vi "TLB Native Dynamic Events ver 0.06a.vi"() -> ()   [LabVIEW 2018]
uses:
  Labview Training Phase 2/Enum Controls/States for Action Engine.ctl
  Type def/TLB event states.ctl
  Type def/TLB MHL States.ctl
  <vilib>/Studica/Studica Toolkit/Background/I2C Channel.ctl
  <vilib>/Studica/Studica Toolkit/NavX/NavX.lvlib
  <vilib>/myRIO/Common/Instrument Driver Framework/myRIO v1.0/AI/typedefs/AI Channels Enum.ctl
  <vilib>/myRIO/Common/Instrument Driver Framework/myRIO v1.0/AI/typedefs/AI Channels List.ctl
  Type def/Type def.ctl
  Type def/Motor Control Cluster.ctl
  <vilib>/Studica/Studica Blackhawk/Blackhawk.lvlib
  <vilib>/vision/driver/NI_Vision_Acquisition_Software.lvlib
  <vilib>/userdefined/High Color/IMAQdx.ctl
  <vilib>/vision/driver/IMAQdx.llb/IMAQdx Buffer Number Mode.ctl
  <vilib>/vision/driver/IMAQdx.llb/IMAQdx Acquisition Mode.ctl
  Underlying VI's/Webcam FGV Low level ver/State control.ctl
  <vilib>/Studica/Studica Toolkit/Background/Mxp Selection.ctl
  <vilib>/ptbypt/NI_PtbyPt.lvlib
panel:
  in  "wTargetSpeed":dbl(slide) scale=-1.0..1.0
  in  "yTargetSpeed":dbl(slide) scale=-1.0..1.0
  in  "xTargetSpeed":dbl(slide) scale=-1.0..1.0
  out "Speed":T1
  out "Distance":T2
  out "Blackhawk loop":i32
  out "NavX Loop":i32
  out "Sensor Loop":i32
  out "User event loop":i32
  out "Event handling loop":i32
  out "Main Loop":i32
  out "Status loop":i32
  out "Waveform Chart 3":dbl(graph)
  out "Waveform Chart 2":dbl(graph)
  out "Waveform Chart":dbl(graph)
  out "L/R average":fxp<+,64,64>
  out "Right Ultrasonic":fxp<+,64,16>
  out "Left Ultrasonic":fxp<+,64,16>
  out "Object detection count":T3
  out "Camera error":errorcluster
  out "Right IR Sensor":dbl
  out "Left IR Sensor":dbl
  in  "Servo Angle":u8(slide) scale=0.0..180.0
  in  "On/Off":bool
  out "Blackhawk error":errorcluster
  out "Value Read":bool
  out "Image Out":T4(plugin-control)
  out "element":T5
  out "Action Queue Items":i32
  out "State Logic Queue Items":i32
  out "Action Queues items":string[](array[string])=["Hardware reset", "Software reset", ""]
  out "State logic":T6=enum."Task 2"
  out "Action State":string
  in  "Tasks Selector":string(combo)="Default"
  out "Yaw":dbl
  out "NavX Info Out":T8
  out "LinearAcceleration":T9
  out "Displacement":T10
  out "YRPHfH":T11
  out "Object detected":bool
  in  "NavX Zero Yaw":bool
  in  "Return to IDLE":bool
  in  "Reset Encoders":bool
  in  "Stop Queue":bool
  in  "Start Task":bool
  # "Camera Status Loop"
  # "TLB FRAMEWORK STATUS"
  # "Test Programme written by Calvin Loke    Dated: 28 Aug 2019\nTest Programme revised by Dr Alex See   Dated 30 Aug 2019\n\nProgramme version:   TLB Native Dynamic Events ver 0.04b.vi"
  # "Sequence of Actions"
  # "Continuous (Repeated)"
  # "Motor Control Loop"
  # "Sensor data"
  # "Blackhawk status"
  # "System Health Status Update"
  # "NAVX Control Loop"
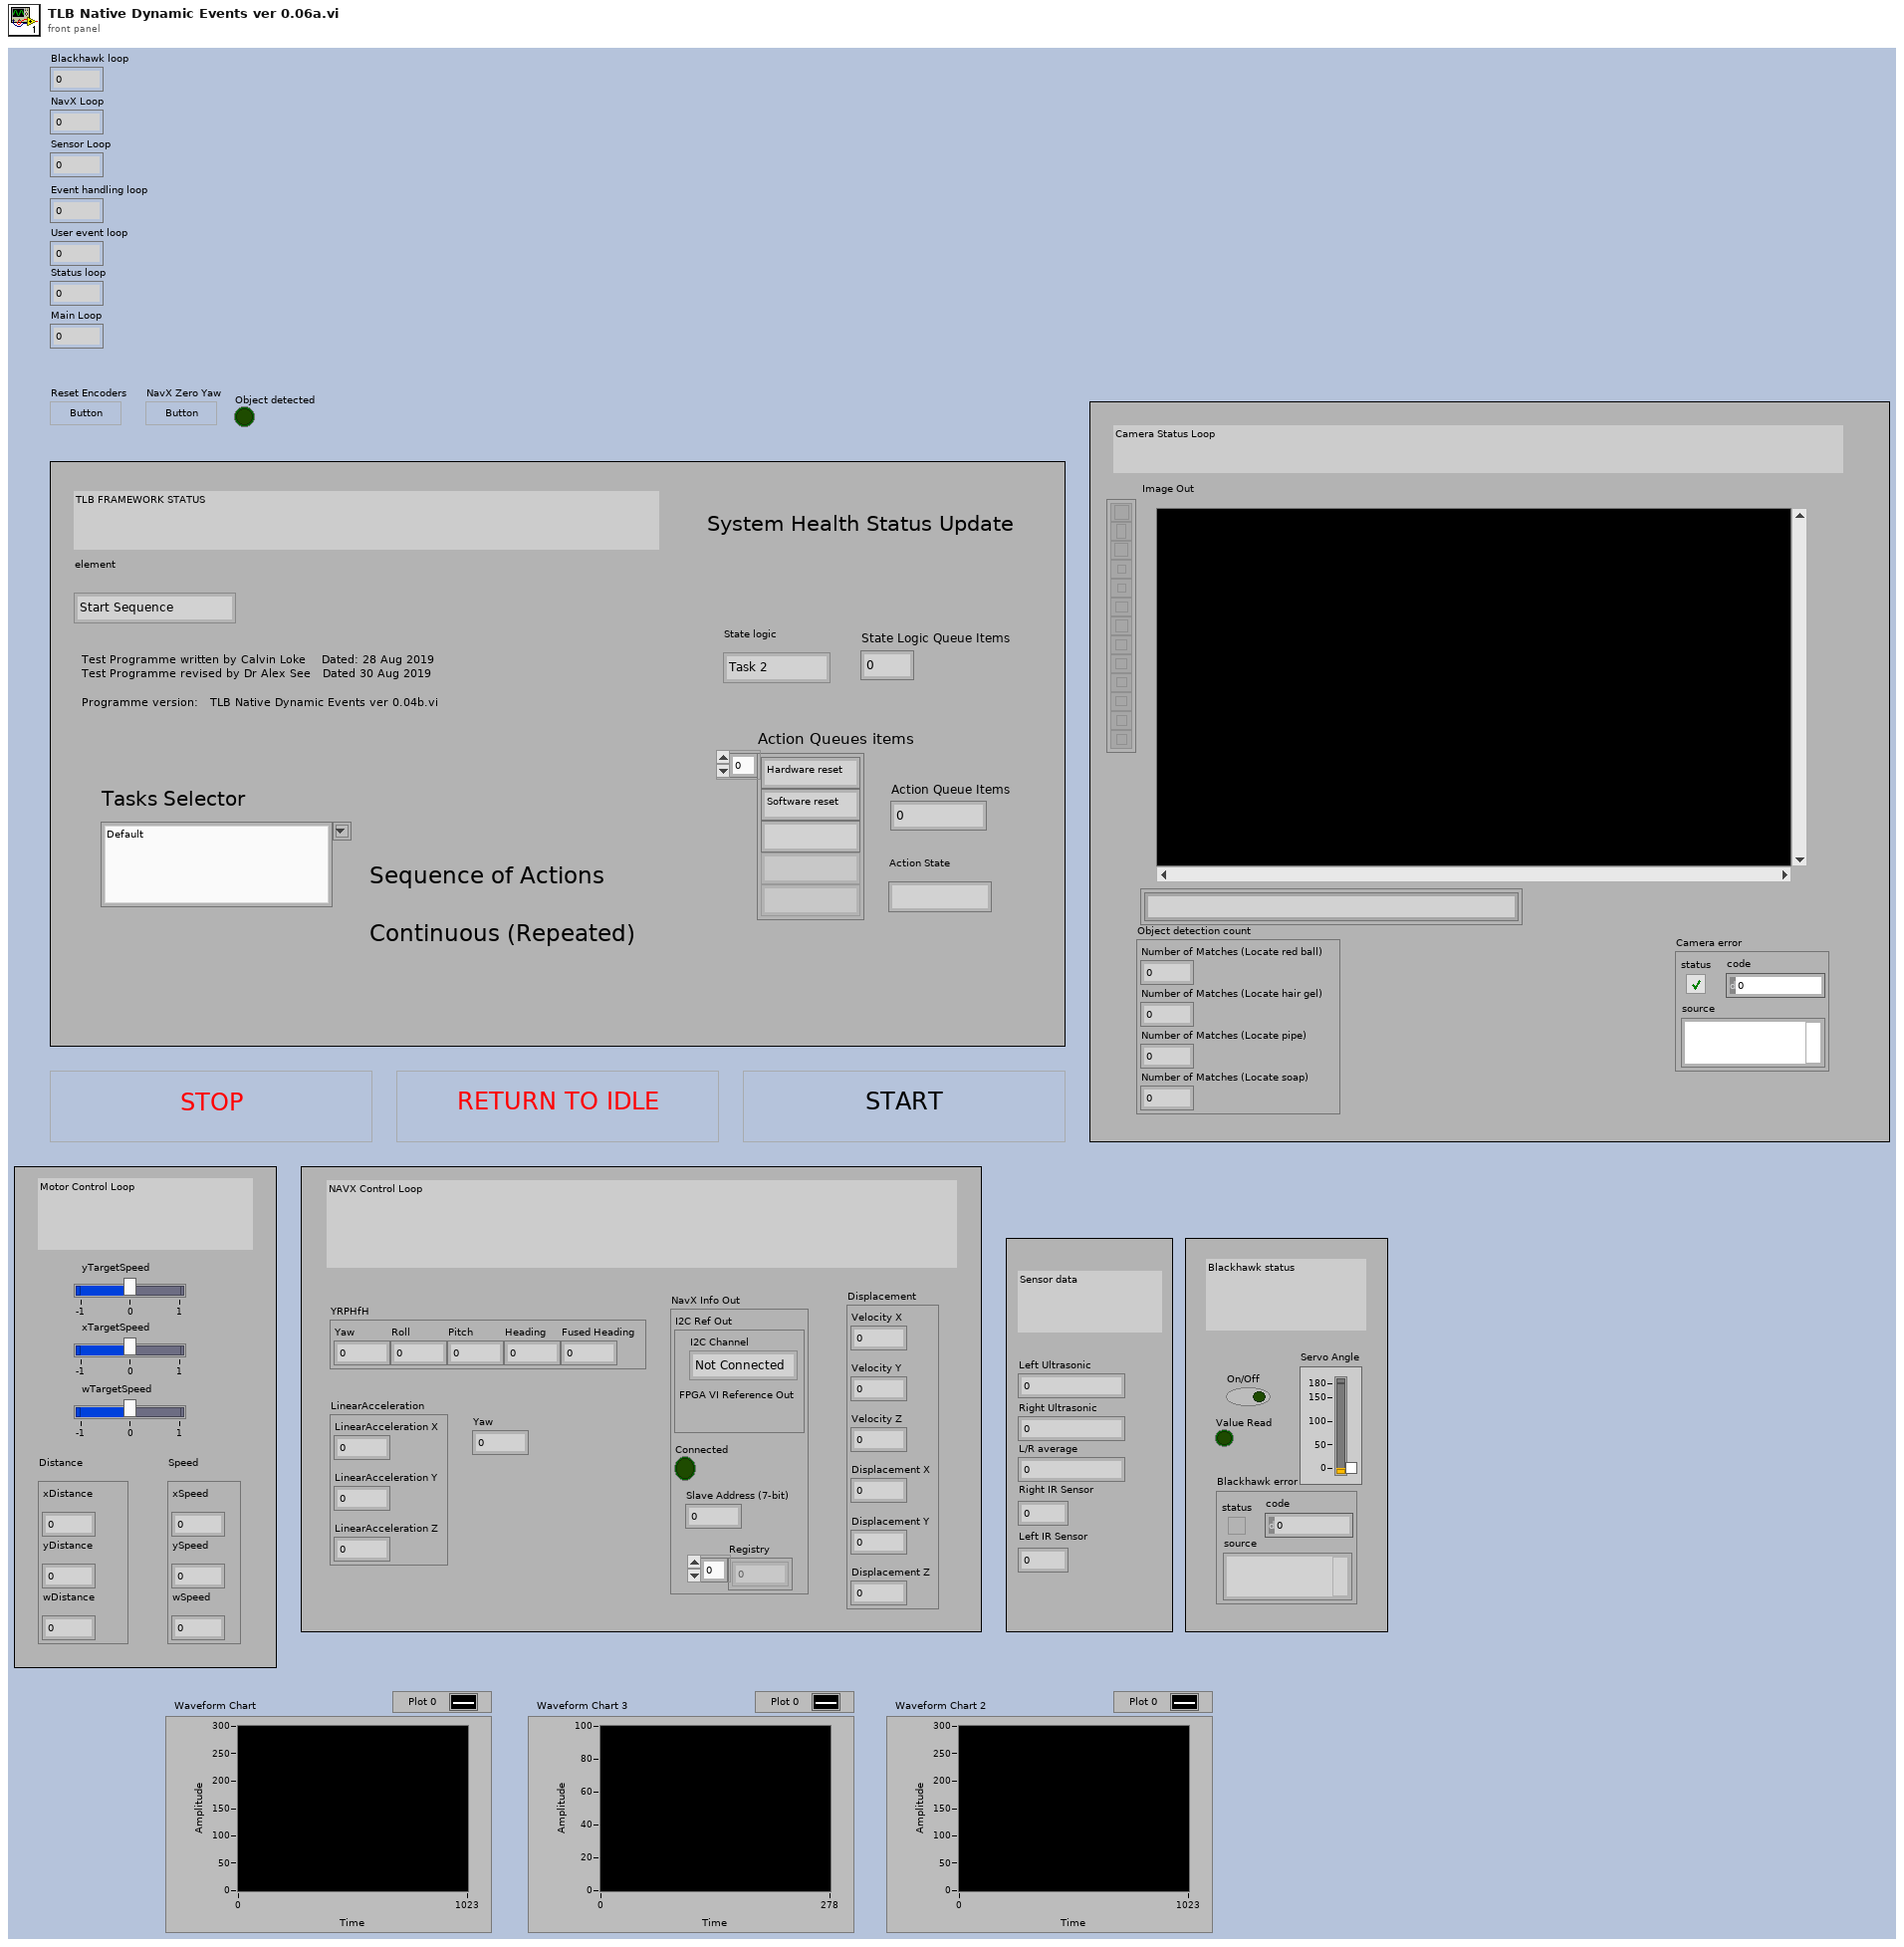
[diagram p1: front panel]
types:
  T1 = cluster{"xSpeed":dbl, "ySpeed":dbl, "wSpeed":dbl}
  T2 = cluster{"xDistance":dbl, "yDistance":dbl, "wDistance":dbl}
  T3 = cluster{"Number of Matches (Locate red ball)":i32, "Number of Matches (Locate hair gel)":i32, "Number of Matches (Locate pipe)":i32, "Number of Matches (Locate soap)":i32}
  T4 = typedef "IMAQ Image.ctl" = refnum<image>
  T5 = typedef "TLB event states.ctl" = enum16{"Start Sequence", "Exit", "Start Task 1", "Start Task 2", "Start Task 3", "Start Task 4", "Camera vision", "Wall follow mode", "Idle", "Start Drive Straight"}
  T6 = typedef "TLB MHL States.ctl" = enum16{"None", "Startup", "Idle", "Processing", "Shutdown", "Reset", "Task 1", "Task 2", "Task 3", "Task 4", "Task 4a", "Task 4b", "Task 4c", "Task 4d", "Task 4e", "Task 4f", "Task 4g", "Task 4h", "Acquire image", "Wall follow mode", "Autodrive", "Autodrive a"}
  T7 = typedef "I2C Channel.ctl" = enum16{"Not Connected", "A", "B"}
  T8 = cluster{"I2C Ref Out":cluster{"I2C Channel":T7, "FPGA VI Reference Out":refnum<k20>}, "Connected":bool, "Slave Address (7-bit)":u8, "Registry":u8[]}
  T9 = cluster{"LinearAcceleration X":dbl, "LinearAcceleration Y":dbl, "LinearAcceleration Z":dbl}
  T10 = cluster{"Velocity X":dbl, "Velocity Y":dbl, "Velocity Z":dbl, "Displacement X":dbl, "Displacement Y":dbl, "Displacement Z":dbl}
  T11 = cluster{"Yaw":dbl, "Roll":dbl, "Pitch":dbl, "Heading":dbl, "Fused Heading":dbl}
  T12 = typedef "States for Action Engine.ctl" = enum16{"Initialize", "Write", "Read"}
  T13 = typedef "Motor Control Cluster.ctl" = cluster{"Vx":dbl, "Vy":dbl, "Vw":dbl}
  T14 = typedef "Type def.ctl" = cluster{"Front Ultrasonic Obstruct":bool, "Left Ultrasonic Obstruct":bool, "Right Ultrasonic Obstruct ":bool}
  T15 = typedef "NI_Vision_Acquisition_Software.lvlib/IMAQdx Acquisition Mode.ctl" = enum32{"One Shot", "Continuous"}
  T16 = typedef "IMAQdx.ctl" = refnum<k21>
  T17 = typedef "NI_Vision_Acquisition_Software.lvlib/IMAQdx Buffer Number Mode.ctl" = enum32{"Next", "Last", "Buffer Number", "Every", "Last New"}
  T18 = typedef "Mxp Selection.ctl" = enum16{"MXP A", "MXP B"}
  T19 = typedef "State control.ctl" = enum16{"Initialise", "Start camera", "Continuous Acquisition ", "Stop camera", "Dispose all"}
  T20 = typedef "AI Channels List.ctl" = T21[]
  T21 = typedef "AI Channels Enum.ctl" = enum16{"Not Connected", "AudioIn/Left", "AudioIn/Right", "C/AI0", "C/AI1", "A/AI0", "A/AI1", "A/AI2", "A/AI3", "A/AI4", "A/AI5", "A/AI6", "A/AI7", "B/AI0", "B/AI1", "B/AI2", "B/AI3", "B/AI4", "B/AI5", "B/AI6", "B/AI7", "AI/AI0", "AI/AI1", "AI/AI2", "AI/AI3", "A/AI0 (DIFF)", "A/AI1 (DIFF)", "A/AI2 (DIFF)", "A/AI3 (DIFF)", "B/AI0 (DIFF)", "B/AI1 (DIFF)", "B/AI2 (DIFF)", "B/AI3 (DIFF)"}
  T22 = cluster{"I2C Channel":T7, "FPGA VI Reference Out":refnum<k20>}
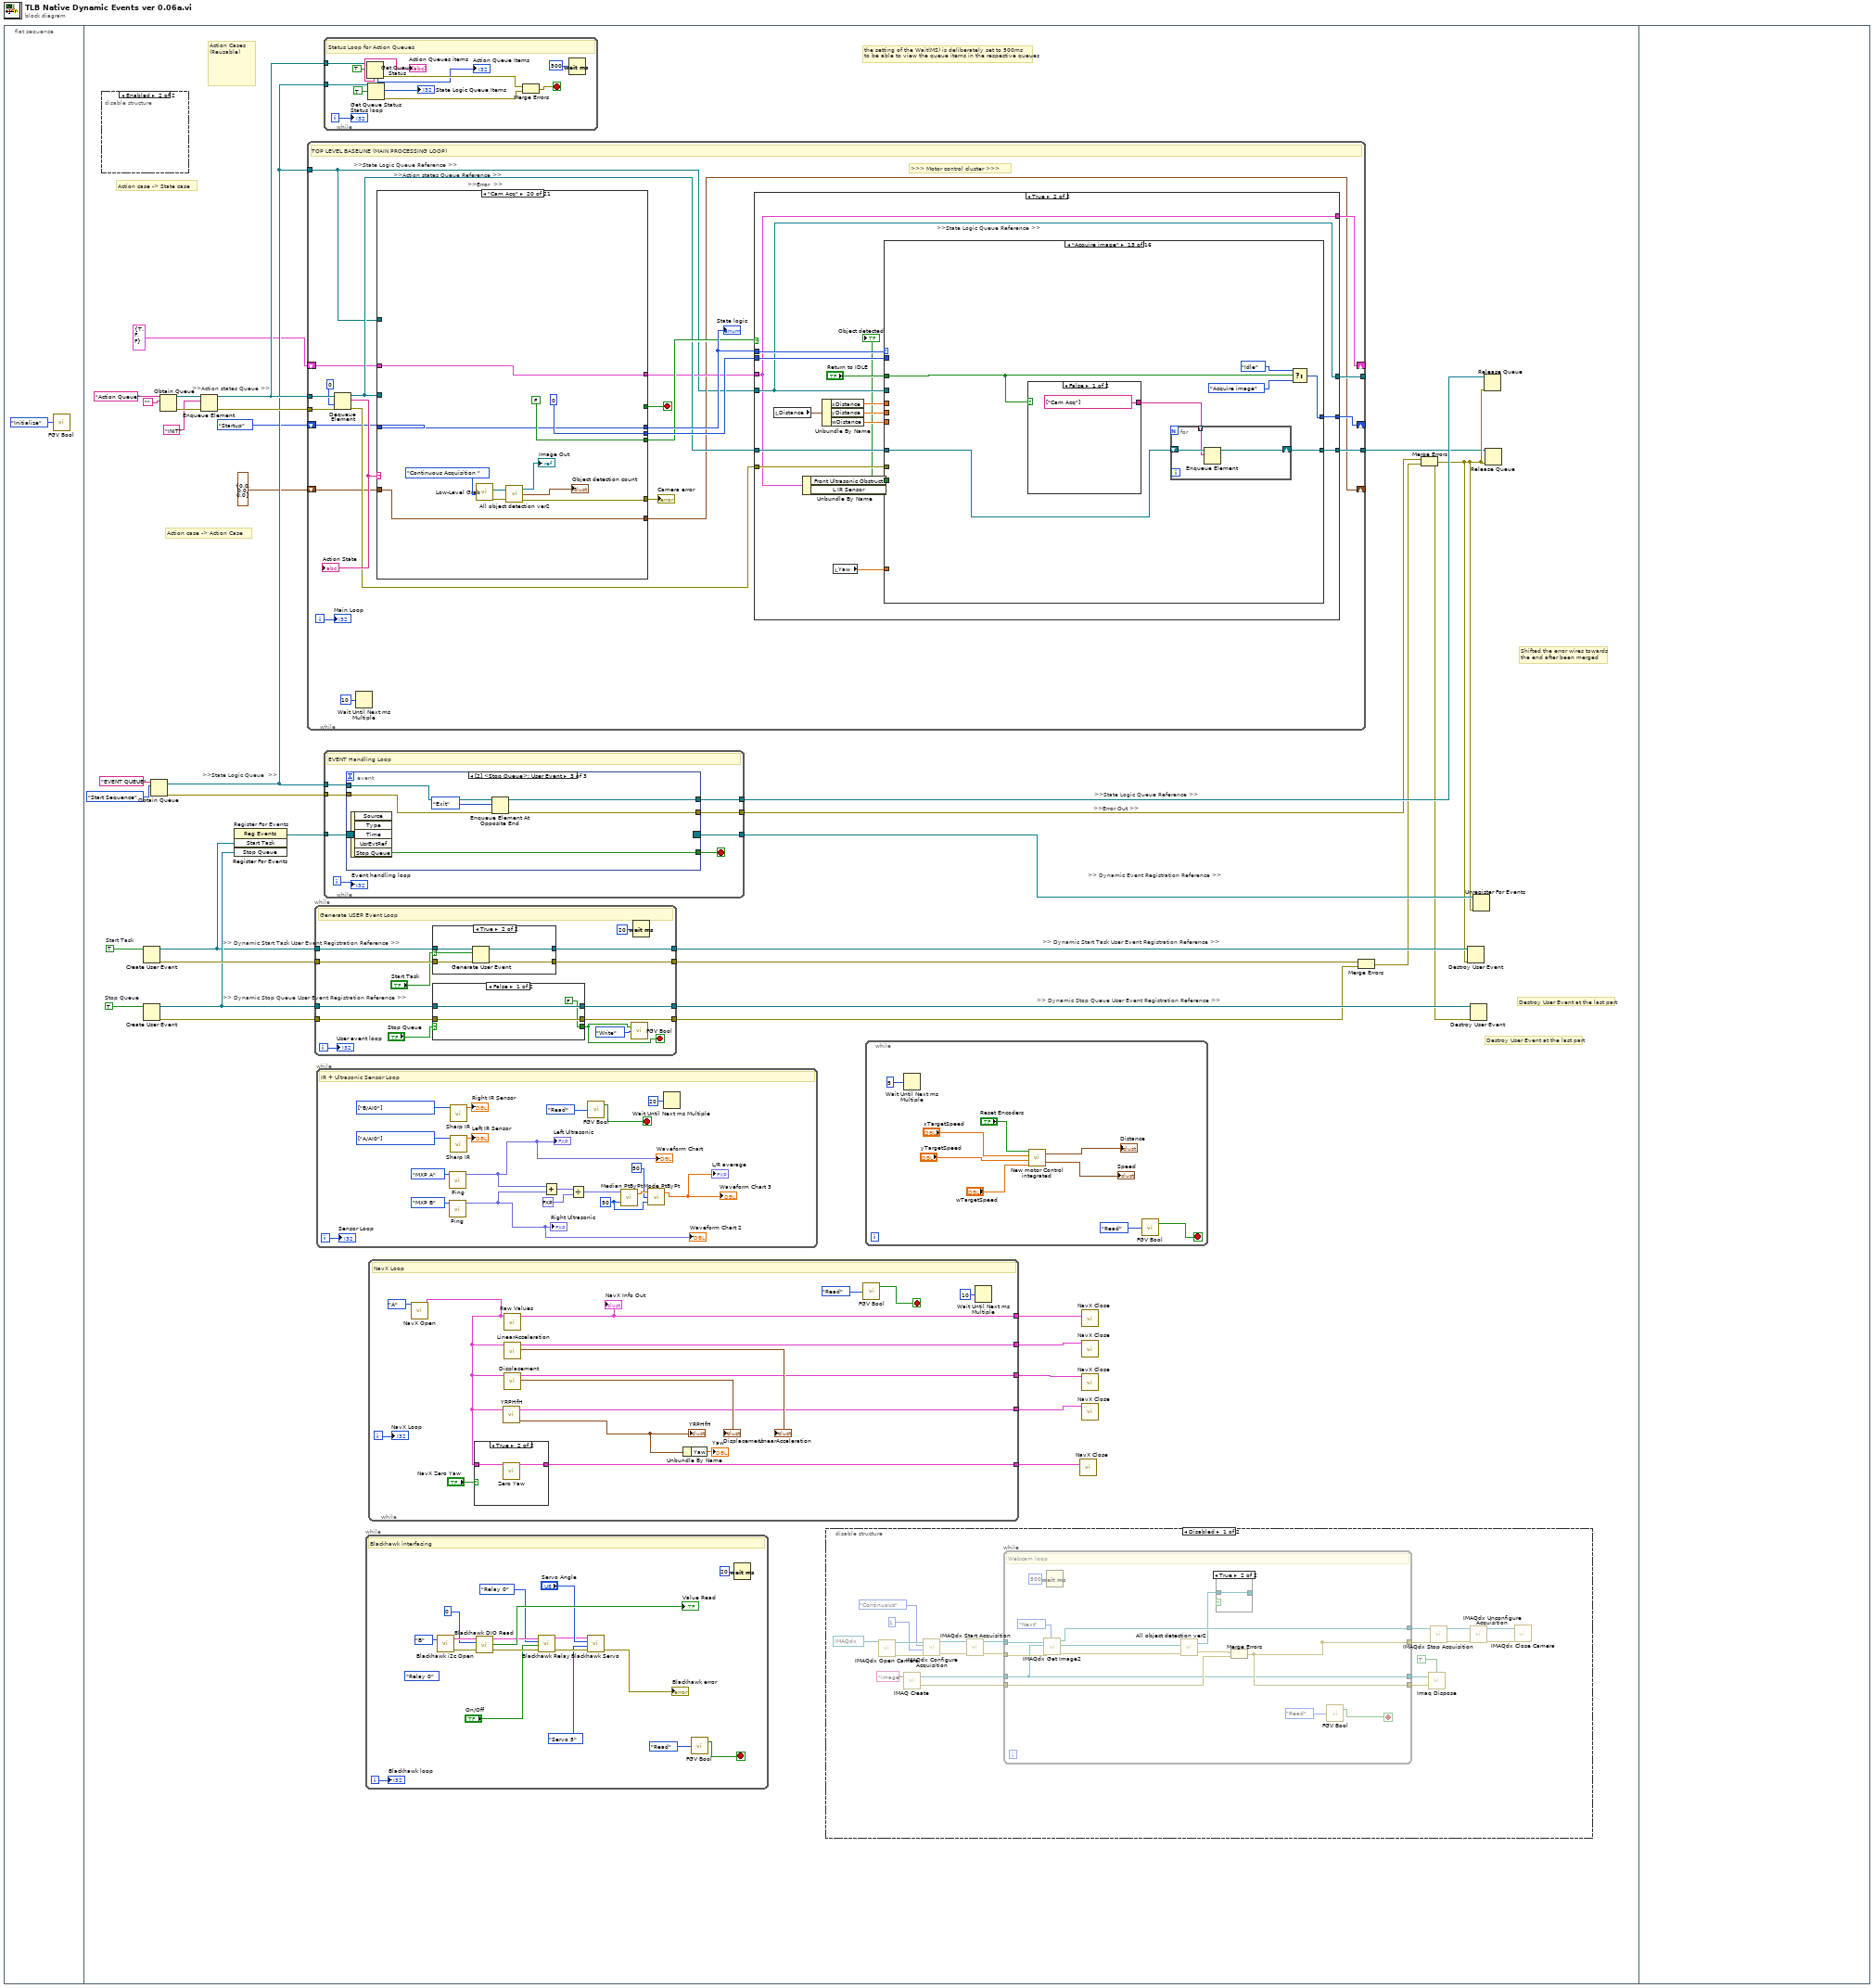
[diagram p0: block diagram]
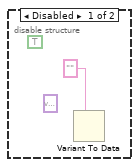
[diagram p5: hidden frame]
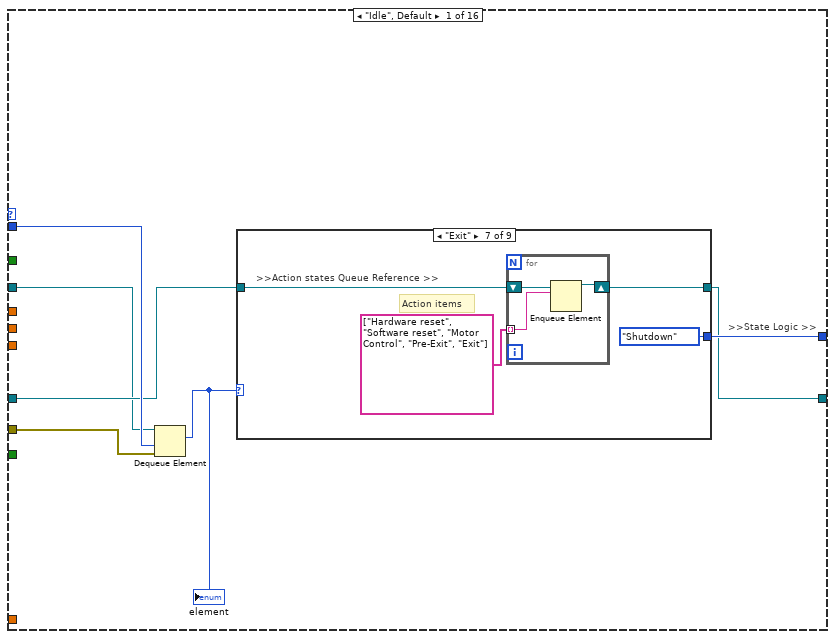
[diagram p7: hidden frame]
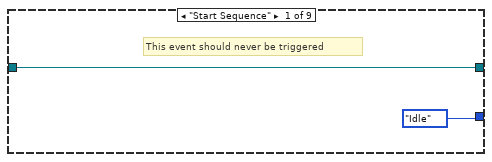
[diagram p8: hidden frame]
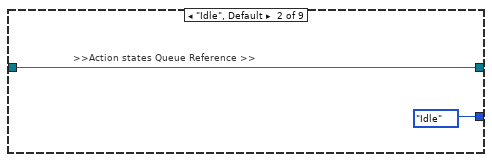
[diagram p9: hidden frame]
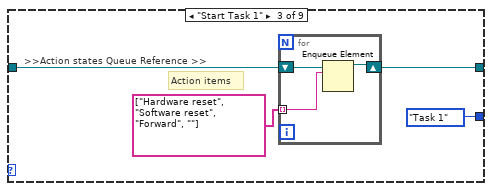
[diagram p10: hidden frame]
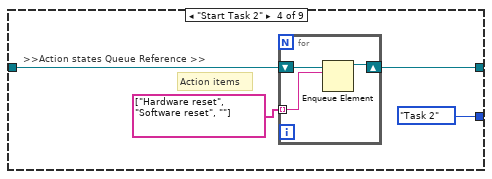
[diagram p11: hidden frame]
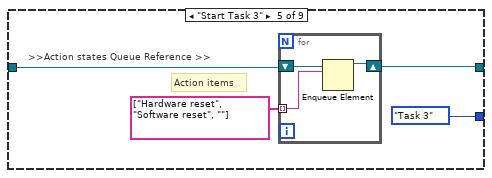
[diagram p12: hidden frame]
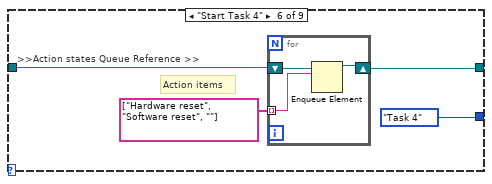
[diagram p13: hidden frame]
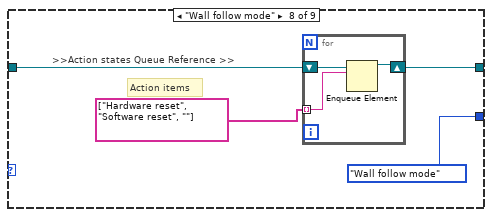
[diagram p14: hidden frame]
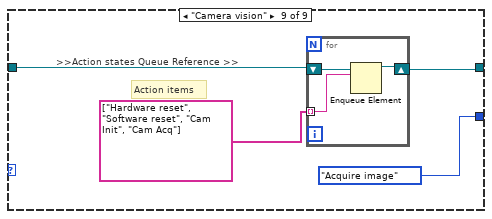
[diagram p15: hidden frame]
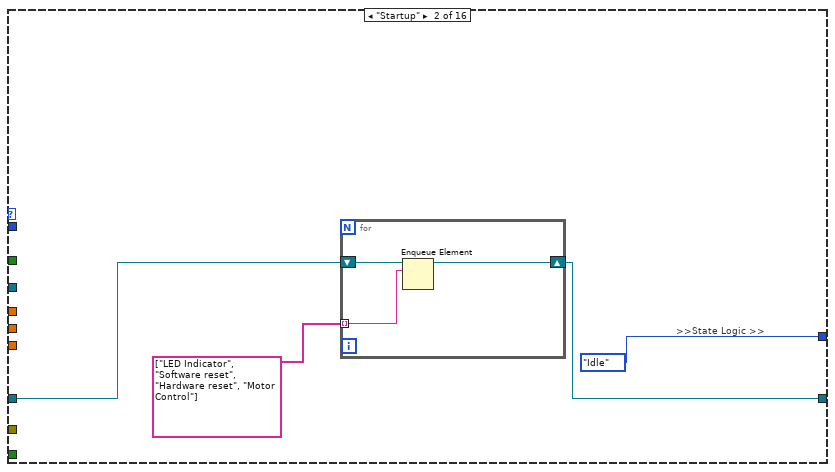
[diagram p16: hidden frame]
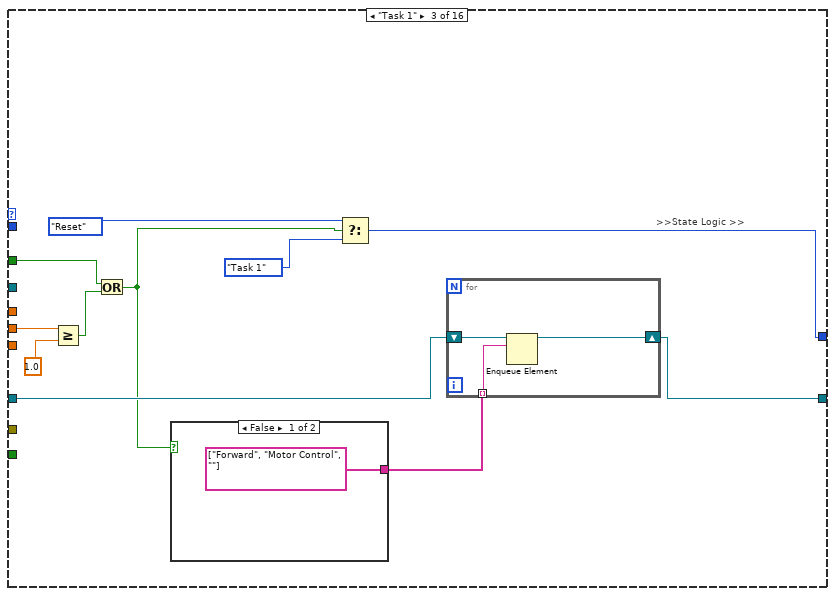
[diagram p17: hidden frame]
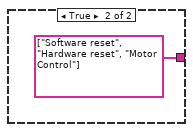
[diagram p18: hidden frame]
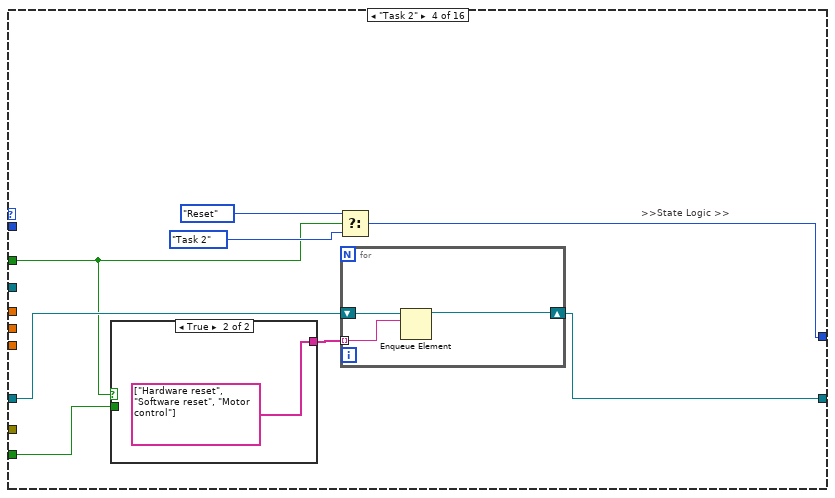
[diagram p19: hidden frame]
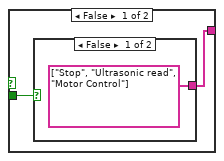
[diagram p20: hidden frame]
diagram:
  n1 = flat-sequence {
    frame #0 {
      n2 = call "FGV Bool.vi"("Init/Read/Write State"=States_for_Action_Engine."Initialize") -> ()  [unwired: 2 in, 2 out]
    }
    frame #1 {
      w37 = TRUE  # Stop Queue
      w36 = TRUE  # Start Task
      # "Action case -> Action Case"
      # "Action case -> State case"
      # "the setting of the Wait(MS) is deliberately set to 500ms\nto be able to view the queue items in the respective queues"
      # "Action Cases\n(Reusable)"
      # ">>Error Out >>"
      # ">> Dynamic Stop Queue User Event Registration Reference >>"
      # ">> Dynamic Start Task User Event Registration Reference >>"
      # ">> Dynamic Stop Queue User Event Registration Reference >>"
      # ">> Dynamic Start Task User Event Registration Reference >>"
      # ">> Dynamic Event Registration Reference >>"
      # ">>Action states Queue >>"
      # ">>State Logic Queue  >>"
      # ">>State Logic Queue Reference >>"
      # "Destroy User Event at the last part"
      # "Destroy User Event at the last part"
      # "Shifted the error wires towards\nthe end after been merged"
      n3 = disable-structure shown="Enabled" {
        frame Disabled {
          (unwired) variant
          (unwired) TRUE
          n4 = Variant To Data(type="") -> ()  [unwired: 2 in, 2 out]
        }
        frame Enabled {
        }
      }
      n5 = Create User Event(user event datatype=w36) -> (user event=w28:refnum<user-event>, error out=w33:errorcluster)  [unwired: 1 in]
      n6 = Create User Event(user event datatype=w37) -> (user event=w29:refnum<user-event>, error out=w32:errorcluster)  [unwired: 1 in]
      n7 = Obtain Queue(name (unnamed)="EVENT QUEUE", element data type=TLB_event_states."Start Sequence" ("Enum")) -> (queue out=w13:refnum<queue>, error out=w19:errorcluster)  [unwired: 3 in, 1 out]
      n8 = Obtain Queue(name (unnamed)="Action Queue", element data type="") -> (queue out=w22:refnum<queue>, error out=w18:errorcluster)  [unwired: 3 in, 1 out]
      n9 = Enqueue Element(queue=w22, element="INIT", error in (no error)=w18) -> (queue out=w14:refnum<queue>, error out=w17:errorcluster)  [unwired: 1 in, 1 out]
      n10 = register-events "Register For Events"(w28, w29) -> (reference out=w27:refnum<event-registration>)  [unwired: 2 in, 1 out]
      n11 = while {
        tunnel: w13 -> [w154]
        shift-right: [w169] -> _
        shift-left: TLB_MHL_States."Startup" ("Enum") -> [w162]
        tunnel: w14 -> [w174]
        tunnel: w17 -> [w172]
        tunnel: [w171] -> _
        tunnel: [w170] -> w11
        shift-right: [w159] -> _
        shift-left: T14 {"Front Ultrasonic Obstruct"=TRUE, "Left Ultrasonic Obstruct"=FALSE, "Right Ultrasonic Obstruct "=FALSE} -> [w161]
        shift-right: [w157] -> _
        shift-left: T13 {"Vx"=0.0, "Vy"=0.0, "Vw"=0.0} -> [w158]
        i -> [w155]
        stop <- w167 stop-if-true
        # ">>> Motor control cluster >>>"
        # ">>Error  >>"
        # ">>Action states Queue Reference >>"
        # ">>State Logic Queue Reference >>"
        # "TOP LEVEL BASELINE (MAIN PROCESSING LOOP)"
        n12 = Dequeue Element(queue=w174, timeout in ms (-1)=0, error in (no error)=w172) -> (queue out=w163:refnum<queue>, element=w173:string, error out=w164:errorcluster)  [unwired: 1 out]
        "Action State" <- w173
        n13 = Wait Until Next ms Multiple(millisecond multiple=u32 10) -> ()  [unwired: 1 out]
        n14 = case shown="\"Cam Acq\"" w173 {
          tunnel: [w420 w437 w442 w450 w459 w469 w478 w485 w496 w504 w512 w522 w532 TLB_MHL_States."Shutdown" ("Enum") w542 w552 w556 w570 w582 w591 w605] -> w175
          tunnel: [w427 0 0 0 0 0 0 0 0 0 0 0 0 0 0 0 0 0 0 0 0] -> w168
          tunnel: [_ _ _ _ _ _ _ _ _ _ _ _ _ TRUE _ _ _ _ _ _ _] -> w167
          tunnel: [TRUE FALSE FALSE FALSE FALSE FALSE FALSE FALSE FALSE FALSE FALSE FALSE FALSE FALSE FALSE FALSE FALSE FALSE FALSE FALSE FALSE] -> w166
          tunnel: w163 -> [w419 _ _ _ _ _ _ _ _ _ _ _ _ _ _ _ _ _ _ _ _]
          tunnel: w162 -> [w421 w437 w442 w450 w459 w469 w478 w485 w496 w504 w512 w522 w532 _ w542 w552 w556 w570 w582 w591 w605]
          tunnel: w161 -> [w425 w434 w439 w446 w455 w464 w473 w482 w491 w500 w513 w519 w527 w534 w543 w551 w559 w571 w583 w590 w601]
          tunnel: [w425 w434 w439 w446 w455 w464 w473 w482 w491 w500 w513 w518 w527 w534 w543 w548 w558 w571 w583 w590 w601] -> w160
          tunnel: w158 -> [w424 w433 w438 w444 w453 w462 w472 w480 w490 w498 w509 w516 w526 w533 w539 w545 w553 w562 w581 w594 w602]
          tunnel: [w424 w433 w438 w445 w454 w463 w471 w481 w489 w499 w509 w516 w524 w533 w539 w545 w553 w563 w581 w594 w602] -> w157
          tunnel: [_ _ _ _ _ _ _ _ _ _ _ _ _ _ _ _ _ _ w572 w586 w595] -> w156
          tunnel: w154 -> [w423 _ _ _ _ _ _ _ _ _ _ _ _ _ _ _ _ _ _ _ _]
          frame "No action", Default {
            n15 = Get Queue Status(queue=w423) -> (error out=w422:errorcluster)  [unwired: 2 in, 7 out]
            n16 = case shown="Error" w422 {
              tunnel: w421 -> [w428 _]
              tunnel: [w428 TLB_MHL_States."Shutdown" ("Enum")] -> w420
              tunnel: w419 -> [_ _]
              frame No Error {
              }
              frame Error {
              }
            }
            n17 = case shown="\"Startup\", Default" w421 {
              tunnel: [0 100] -> w427
              frame "Startup", Default {
              }
              frame "Idle" {
              }
            }
          }
          frame "Init" {
            # ">>State Logic  >>"
            n18 = local write "Servo Angle"(u8 90 ("Servo Angle")) -> ()
          }
          frame "LED Indicator" {
          }
          frame "Forward" {
            n19 = local write "NavX Zero Yaw"(FALSE ("NavX Zero Yaw")) -> ()
            n20 = local write "Reset Encoders"(FALSE ("Reset Encoder 0")) -> ()
            n21 = Bundle By Name(cluster=w444, "Vy"=0.6) -> (w445:T13)
          }
          frame "Reverse" {
            n22 = local write "NavX Zero Yaw"(FALSE ("NavX Zero Yaw")) -> ()
            n23 = local write "Reset Encoders"(FALSE ("Reset Encoder 0")) -> ()
            n24 = Bundle By Name(cluster=w453, "Vy"=-0.6) -> (w454:T13)
          }
          frame "Right" {
            n25 = local write "NavX Zero Yaw"(FALSE ("NavX Zero Yaw")) -> ()
            n26 = local write "Reset Encoders"(FALSE ("Reset Encoder 0")) -> ()
            n27 = Bundle By Name(cluster=w462, "Vx"=0.6) -> (w463:T13)
          }
          frame "Left" {
            n28 = Bundle By Name(cluster=w472, "Vx"=-0.6) -> (w471:T13)
            n29 = local write "NavX Zero Yaw"(FALSE ("NavX Zero Yaw")) -> ()
            n30 = local write "Reset Encoders"(FALSE ("Reset Encoder 0")) -> ()
          }
          frame "Rotate CW" {
            n31 = local write "NavX Zero Yaw"(FALSE ("NavX Zero Yaw")) -> ()
            n32 = local write "Reset Encoders"(FALSE ("Reset Encoder 0")) -> ()
            n33 = Bundle By Name(cluster=w480, "Vw"=-0.3) -> (w481:T13)
          }
          frame "Rotate ACW" {
            n34 = local write "Reset Encoders"(FALSE ("Reset Encoder 0")) -> ()
            n35 = local write "NavX Zero Yaw"(FALSE ("NavX Zero Yaw")) -> ()
            n36 = Bundle By Name(cluster=w490, "Vw"=0.15) -> (w489:T13)
          }
          frame "Stop" {
            w497 = 0.0
            n37 = local write "NavX Zero Yaw"(FALSE ("NavX Zero Yaw")) -> ()
            n38 = local write "Reset Encoders"(FALSE ("Reset Encoder 0")) -> ()
            n39 = Bundle By Name(cluster=w498, "Vx"=w497, "Vy"=w497, "Vw"=w497) -> (w499:T13)
          }
          frame "Motor control" {
            # "Replace with FGV"
            n40 = Unbundle By Name(w509) -> ("Vx"=w508:dbl, "Vy"=w507:dbl, "Vw"=w506:dbl)
            n41 = local write "xTargetSpeed"(w508) -> ()
            n42 = local write "yTargetSpeed"(w507) -> ()
            n43 = local write "wTargetSpeed"(w506) -> ()
          }
          frame "Software reset" {
            w517 = FALSE ("NavX Zero Yaw")
            n44 = Wait (ms)(milliseconds to wait=u32 20) -> ()  [unwired: 1 out]
            n45 = local write "NavX Zero Yaw"(w517) -> ()
            n46 = Bundle By Name(cluster=w519, "Front Ultrasonic Obstruct"=w517, "L IR Sensor"=0.0) -> (w518:T14)
          }
          frame "Hardware reset" {
            w525 = 0.0
            n47 = Wait (ms)(milliseconds to wait=u32 20) -> ()  [unwired: 1 out]
            n48 = local write "NavX Zero Yaw"(TRUE ("NavX Zero Yaw")) -> ()
            n49 = local write "Reset Encoders"(TRUE ("Reset Encoder 0")) -> ()
            n50 = Bundle By Name(cluster=w526, "Vx"=w525, "Vy"=w525, "Vw"=w525) -> (w524:T13)
          }
          frame "Exit" {
          }
          frame "Pre-Exit" {
          }
          frame "Ultrasonic read" {
            # "Object detection"
            n51 = local read "L/R average"() -> (w544:fxp<+,64,64>)
            n52 = Less Or Equal?(x=w544, y=35.0) -> (x <= y?=w546:bool)
            n53 = Bundle By Name(cluster=w551, "Front Ultrasonic Obstruct"=w546) -> (w548:T14)
          }
          frame "IR Sensor Read" {
            n54 = local read "Left IR Sensor"() -> (w557:dbl)
            n55 = Bundle By Name(cluster=w559, "L IR Sensor"=w557) -> (w558:T14)
          }
          frame "Calculate" {
            n56 = Unbundle By Name(w571) -> ("L IR Sensor"=w567:dbl)
            n57 = Subtract(x=w567, y=20.0) -> (x-y=w565:dbl)
            n58 = Multiply(x=w565, y=0.01) -> (x*y=w561:dbl)
            n59 = Bundle By Name(cluster=w562, "Vy"=0.4, "Vw"=w561) -> (w563:T13)
          }
          frame "Cam Init" {
            n60 = call "Low-Level Grab.vi"("States"=State_control."Initialise", "Session In"=T16 "cam1") -> ("error out"=w573:errorcluster, "Session Out"=w574:T16)  [unwired: 7 in, 1 out]
            n61 = call "Low-Level Grab.vi"("error in (no error)"=w573, "States"=State_control."Start camera", "Session In"=w574) -> ("error out"=w572:errorcluster)  [unwired: 6 in, 2 out]
            n62 = local write "Servo Angle"(u8 170 ("Servo Angle")) -> ()
          }
          frame "Cam Acq" {
            n63 = call "Low-Level Grab.vi"("States"=State_control."Continuous Acquisition ") -> ("error out"=w587:errorcluster, "Image Out"=w588:T4)  [unwired: 8 in, 1 out]
            n64 = call "All object detection ver2.vi"("Image In"=w588, "error in"=w587) -> ("Image Out"=→"Image Out":T4, "Object detection count"=→"Object detection count":T3, "error out"=w586:errorcluster)
          }
          frame "Cam Exit" {
            n65 = call "Low-Level Grab.vi"("States"=State_control."Stop camera") -> ("error out"=w596:errorcluster, "Session Out"=w598:T16)  [unwired: 8 in, 1 out]
            n66 = local write "Servo Angle"(u8 90 ("Servo Angle")) -> ()
            n67 = call "Low-Level Grab.vi"("error in (no error)"=w596, "States"=State_control."Dispose all", "Session In"=w598) -> ("error out"=w595:errorcluster)  [unwired: 6 in, 2 out]
          }
        }
        "State logic" <- w175
        "Camera error" <- w156
        n68 = case shown="True" w166 {
          tunnel: w175 -> [w178 w194]
          tunnel: w154 -> [w179 w188]
          tunnel: w163 -> [w177 w193]
          tunnel: [w179 w188] -> w171
          tunnel: [w177 w192] -> w170
          tunnel: [w178 w191] -> w169
          tunnel: w164 -> [_ w190]
          tunnel: w168 -> [_ w189]
          tunnel: w160 -> [w176 w181]
          tunnel: [w176 w181] -> w159
          frame False {
          }
          frame True {
            # ">>State Logic Queue Reference >>"
            n69 = local read "Distance"() -> (w180:T2)
            n70 = Unbundle By Name(w181) -> ("Front Ultrasonic Obstruct"=w182:bool)  [unwired: 1 out]
            "Object detected" <- w182
            n71 = Unbundle By Name(w180) -> ("xDistance"=w184:dbl, "yDistance"=w186:dbl, "wDistance"=w185:dbl)
            n72 = local read "Yaw"() -> (w183:dbl)
            n73 = case shown="\"Acquire image\"" w194 {
              tunnel: w188 -> [w195 _ _ _ _ _ _ _ _ _ _ _ _ _ _ _]
              tunnel: w193 -> [w197 w256 w268 w281 w303 w312 w326 w341 w354 w367 w378 w386 w399 w408 w411 w417]
              tunnel: [w196 w255 w267 w282 w302 w313 w325 w340 w353 w366 w377 w387 w398 w408 w410 w417] -> w192
              tunnel: [w200 TLB_MHL_States."Idle" ("Enum") w270 w283 w299 w316 w328 w339 w355 w365 TLB_MHL_States."Idle" ("Enum") w389 w397 TLB_MHL_States."Reset" ("Enum") TLB_MHL_States."Shutdown" ("Enum") TLB_MHL_States."Reset" ("Enum")] -> w191
              tunnel: w190 -> [w198 _ _ _ _ _ _ _ _ _ _ _ _ _ _ _]
              tunnel: w189 -> [w199 _ _ _ _ _ _ _ _ _ _ _ _ _ _ _]
              tunnel: "Return to IDLE" -> [_ _ w265 w280 w297 _ _ _ _ _ _ w384 w396 _ _ _]
              tunnel: w186 -> [_ _ w262 _ _ _ w322 w336 _ _ _ _ _ _ _ _]
              tunnel: w185 -> [_ _ _ _ w294 _ _ _ _ _ _ _ _ _ _ _]
              tunnel: w184 -> [_ _ _ _ _ _ _ _ w350 _ _ _ _ _ _ _]
              tunnel: w183 -> [_ _ _ _ _ _ _ _ _ _ _ _ _ _ _ _]
              tunnel: w182 -> [_ _ _ w278 _ w310 _ _ _ w364 _ _ _ _ _ _]
              frame "Idle", Default {
                # ">>State Logic >>"
                n74 = Dequeue Element(queue=w195, timeout in ms (-1)=w199, error in (no error)=w198) -> (element=w201:T5)  [unwired: 3 out]
                "element" <- w201
                n75 = case shown="\"Exit\"" w201 {
                  tunnel: [TLB_MHL_States."Idle" ("Enum") TLB_MHL_States."Idle" ("Enum") TLB_MHL_States."Task 1" ("Enum") TLB_MHL_States."Task 2" ("Enum") TLB_MHL_States."Task 3" ("Enum") TLB_MHL_States."Task 4" ("Enum") TLB_MHL_States."Shutdown" ("Enum") TLB_MHL_States."Wall follow mode" ("Enum") TLB_MHL_States."Acquire image" ("Enum")] -> w200
                  tunnel: [w203 w204 w208 w213 w222 w228 w234 w241 w249] -> w196
                  tunnel: w197 -> [w203 w204 w206 w214 w223 w229 w235 w242 w250]
                  frame "Start Sequence" {
                    # "This event should never be triggered"
                  }
                  frame "Idle", Default {
                    # ">>Action states Queue Reference >>"
                  }
                  frame "Start Task 1" {
                    # ">>Action states Queue Reference >>"
                    # "Action items"
                    n76 = for {
                      shift-right: [w212] -> w208
                      shift-left: w206 -> [w211]
                      tunnel: string[] ["Hardware reset", "Software reset", "Forward", ""] -> [w210] mode=indexing
                      n77 = Enqueue Element(queue=w211, element=w210) -> (queue out=w212:refnum<queue>)  [unwired: 2 in, 2 out]
                    }
                  }
                  frame "Start Task 2" {
                    # ">>Action states Queue Reference >>"
                    # "Action items"
                    n78 = for {
                      shift-right: [w219] -> w213
                      shift-left: w214 -> [w218]
                      tunnel: string[] ["Hardware reset", "Software reset", ""] -> [w217] mode=indexing
                      n79 = Enqueue Element(queue=w218, element=w217) -> (queue out=w219:refnum<queue>)  [unwired: 2 in, 2 out]
                    }
                  }
                  frame "Start Task 3" {
                    # ">>Action states Queue Reference >>"
                    # "Action items"
                    n80 = for {
                      shift-right: [w226] -> w222
                      shift-left: w223 -> [w225]
                      tunnel: string[] ["Hardware reset", "Software reset", ""] -> [w224] mode=indexing
                      n81 = Enqueue Element(queue=w225, element=w224) -> (queue out=w226:refnum<queue>)  [unwired: 2 in, 2 out]
                    }
                  }
                  frame "Start Task 4" {
                    # ">>Action states Queue Reference >>"
                    # "Action items"
                    n82 = for {
                      shift-right: [w233] -> w228
                      shift-left: w229 -> [w232]
                      tunnel: string[] ["Hardware reset", "Software reset", ""] -> [w231] mode=indexing
                      n83 = Enqueue Element(queue=w232, element=w231) -> (queue out=w233:refnum<queue>)  [unwired: 2 in, 2 out]
                    }
                  }
                  frame "Exit" {
                    # ">>Action states Queue Reference >>"
                    # "Action items"
                    n84 = for {
                      shift-right: [w240] -> w234
                      shift-left: w235 -> [w239]
                      tunnel: string[] ["Hardware reset", "Software reset", "Motor Control", "Pre-Exit", "Exit"] -> [w238] mode=indexing
                      n85 = Enqueue Element(queue=w239, element=w238) -> (queue out=w240:refnum<queue>)  [unwired: 2 in, 2 out]
                    }
                  }
                  frame "Wall follow mode" {
                    # ">>Action states Queue Reference >>"
                    # "Action items"
                    n86 = for {
                      shift-right: [w247] -> w241
                      shift-left: w242 -> [w246]
                      tunnel: string[] ["Hardware reset", "Software reset", ""] -> [w245] mode=indexing
                      n87 = Enqueue Element(queue=w246, element=w245) -> (queue out=w247:refnum<queue>)  [unwired: 2 in, 2 out]
                    }
                  }
                  frame "Camera vision" {
                    # ">>Action states Queue Reference >>"
                    # "Action items"
                    n88 = for {
                      shift-right: [w254] -> w249
                      shift-left: w250 -> [w253]
                      tunnel: string[] ["Hardware reset", "Software reset", "Cam Init", "Cam Acq"] -> [w252] mode=indexing
                      n89 = Enqueue Element(queue=w253, element=w252) -> (queue out=w254:refnum<queue>)  [unwired: 2 in, 2 out]
                    }
                  }
                }
              }
              frame "Startup" {
                # ">>State Logic >>"
                n90 = for {
                  shift-right: [w260] -> w255
                  shift-left: w256 -> [w261]
                  tunnel: string[] ["LED Indicator", "Software reset", "Hardware reset", "Motor Control"] -> [w259] mode=indexing
                  n91 = Enqueue Element(queue=w261, element=w259) -> (queue out=w260:refnum<queue>)  [unwired: 2 in, 2 out]
                }
              }
              frame "Task 1" {
                # ">>State Logic >>"
                n92 = Greater Or Equal?(x=w262, y=1.0) -> (x >= y?=w263:bool)
                n93 = Or(x=w265, y=w263) -> (x .or. y?=w266:bool)
                n94 = case shown="False" w266 {
                  tunnel: [string[] ["Forward", "Motor Control", ""] string[] ["Software reset", "Hardware reset", "Motor Control"]] -> w269
                  frame False {
                  }
                  frame True {
                  }
                }
                n95 = Select(t=TLB_MHL_States."Reset" ("Enum"), s=w266, f=TLB_MHL_States."Task 1" ("Enum")) -> (s? t:f=w270:T6)
                n96 = for {
                  shift-right: [w276] -> w267
                  shift-left: w268 -> [w277]
                  tunnel: w269 -> [w275] mode=indexing
                  n97 = Enqueue Element(queue=w277, element=w275) -> (queue out=w276:refnum<queue>)  [unwired: 2 in, 2 out]
                }
              }
              frame "Task 2" {
                # ">>State Logic >>"
                n98 = case shown="True" w280 {
                  tunnel: [w287 string[] ["Hardware reset", "Software reset", "Motor control"]] -> w279
                  tunnel: w278 -> [w286 _]
                  frame False {
                    n99 = case shown="False" w286 {
                      tunnel: [string[] ["Stop", "Ultrasonic read", "Motor Control"] string[] ["Reverse", "Ultrasonic read", "Motor control"]] -> w287
                      frame False {
                      }
                      frame True {
                      }
                    }
                  }
                  frame True {
                  }
                }
                n100 = Select(t=TLB_MHL_States."Reset" ("Enum"), s=w280, f=TLB_MHL_States."Task 2" ("Enum")) -> (s? t:f=w283:T6)
                n101 = for {
                  shift-right: [w292] -> w282
                  shift-left: w281 -> [w293]
                  tunnel: w279 -> [w291] mode=indexing
                  n102 = Enqueue Element(queue=w293, element=w291) -> (queue out=w292:refnum<queue>)  [unwired: 2 in, 2 out]
                }
              }
              frame "Task 3" {
                n103 = Less Or Equal?(x=w294, y=-1.2) -> (x <= y?=w295:bool)
                n104 = Or(x=w295, y=w297) -> (x .or. y?=w298:bool)
                n105 = case shown="True" w298 {
                  tunnel: [string[] ["Rotate CW", "Motor Control"] string[] ["Software reset", "Hardware reset", "Motor Control"]] -> w304
                  frame False {
                  }
                  frame True {
                  }
                }
                n106 = for {
                  shift-right: [w306] -> w302
                  shift-left: w303 -> [w307]
                  tunnel: w304 -> [w305] mode=indexing
                  n107 = Enqueue Element(queue=w307, element=w305) -> (queue out=w306:refnum<queue>)  [unwired: 2 in, 2 out]
                }
                n108 = Select(t=TLB_MHL_States."Reset" ("Enum"), s=w298, f=TLB_MHL_States."Task 3" ("Enum")) -> (s? t:f=w299:T6)
              }
              frame "Task 4" {
                n109 = case shown="False" w310 {
                  tunnel: [string[] ["Forward", "Ultrasonic read", "Motor Control"] string[] ["Stop", "Hardware reset", "Software reset", "Motor Control"]] -> w311
                  frame False {
                  }
                  frame True {
                  }
                }
                n110 = for {
                  shift-right: [w320] -> w313
                  shift-left: w312 -> [w321]
                  tunnel: w311 -> [w319] mode=indexing
                  n111 = Enqueue Element(queue=w321, element=w319) -> (queue out=w320:refnum<queue>)  [unwired: 2 in, 2 out]
                }
                n112 = Select(t=TLB_MHL_States."Task 4a" ("Enum"), s=w310, f=TLB_MHL_States."Task 4" ("Enum")) -> (s? t:f=w316:T6)
              }
              frame "Task 4a" {
                n113 = Greater Or Equal?(x=w322, y=0.5) -> (x >= y?=w324:bool)
                n114 = case shown="True" w324 {
                  tunnel: [string[] ["Right", "Motor Control"] string[] ["Stop", "Hardware reset", "Software reset", "Motor Control"]] -> w327
                  frame False {
                  }
                  frame True {
                  }
                }
                n115 = for {
                  shift-right: [w334] -> w325
                  shift-left: w326 -> [w335]
                  tunnel: w327 -> [w333] mode=indexing
                  n116 = Enqueue Element(queue=w335, element=w333) -> (queue out=w334:refnum<queue>)  [unwired: 2 in, 2 out]
                }
                n117 = Select(t=TLB_MHL_States."Task 4b" ("Enum"), s=w324, f=TLB_MHL_States."Task 4a" ("Enum")) -> (s? t:f=w328:T6)
              }
              frame "Task 4b" {
                n118 = Greater Or Equal?(x=w336, y=0.75) -> (x >= y?=w337:bool)
                n119 = case shown="False" w337 {
                  tunnel: [string[] ["Forward", "Motor control"] string[] ["Stop", "Hardware reset", "Software reset"]] -> w342
                  frame False {
                  }
                  frame True {
                  }
                }
                n120 = for {
                  shift-right: [w348] -> w340
                  shift-left: w341 -> [w349]
                  tunnel: w342 -> [w347] mode=indexing
                  n121 = Enqueue Element(queue=w349, element=w347) -> (queue out=w348:refnum<queue>)  [unwired: 2 in, 2 out]
                }
                n122 = Select(t=TLB_MHL_States."Task 4c" ("Enum"), s=w337, f=TLB_MHL_States."Task 4b" ("Enum")) -> (s? t:f=w339:T6)
              }
              frame "Task 4c" {
                n123 = Less Or Equal?(x=w350, y=-0.65) -> (x <= y?=w351:bool)
                n124 = case shown="False" w351 {
                  tunnel: [string[] ["Left"] string[] ["Stop", "Hardware reset", "Software reset"]] -> w356
                  frame False {
                  }
                  frame True {
                  }
                }
                n125 = for {
                  shift-right: [w362] -> w353
                  shift-left: w354 -> [w363]
                  tunnel: w356 -> [w361] mode=indexing
                  n126 = Enqueue Element(queue=w363, element=w361) -> (queue out=w362:refnum<queue>)  [unwired: 2 in, 2 out]
                }
                n127 = Select(t=TLB_MHL_States."Task 4d" ("Enum"), s=w351, f=TLB_MHL_States."Task 4c" ("Enum")) -> (s? t:f=w355:T6)
              }
              frame "Task 4d" {
                n128 = case shown="False" w364 {
                  tunnel: [string[] ["Forward", "Ultrasonic Read"] string[] ["Stop", "Hardware reset", "Software reset"]] -> w368
                  frame False {
                  }
                  frame True {
                  }
                }
                n129 = for {
                  shift-right: [w374] -> w366
                  shift-left: w367 -> [w375]
                  tunnel: w368 -> [w373] mode=indexing
                  n130 = Enqueue Element(queue=w375, element=w373) -> (queue out=w374:refnum<queue>)  [unwired: 2 in, 2 out]
                }
                n131 = Select(t=TLB_MHL_States."Task 4e" ("Enum"), s=w364, f=TLB_MHL_States."Task 4d" ("Enum")) -> (s? t:f=w365:T6)
              }
              frame "Reset" {
                n132 = for {
                  shift-right: [w382] -> w377
                  shift-left: w378 -> [w383]
                  tunnel: string[] ["Software reset", "Hardware reset", ""] -> [w381] mode=indexing
                  n133 = Enqueue Element(queue=w383, element=w381) -> (queue out=w382:refnum<queue>)  [unwired: 2 in, 2 out]
                }
                n134 = Wait (ms)(milliseconds to wait=u32 250) -> ()  [unwired: 1 out]
              }
              frame "Wall follow mode" {
                n135 = case shown="True" w384 {
                  tunnel: [string[] ["IR Sensor Read", "Calculate", "Forward", "Motor Control"] string[] ["Hardware reset", "Software reset", "Motor Control"]] -> w385
                  frame False {
                  }
                  frame True {
                  }
                }
                n136 = for {
                  shift-right: [w394] -> w387
                  shift-left: w386 -> [w395]
                  tunnel: w385 -> [w393] mode=indexing
                  n137 = Enqueue Element(queue=w395, element=w393) -> (queue out=w394:refnum<queue>)  [unwired: 2 in, 2 out]
                }
                n138 = Select(t=TLB_MHL_States."Idle" ("Enum"), s=w384, f=TLB_MHL_States."Wall follow mode" ("Enum")) -> (s? t:f=w389:T6)
              }
              frame "Acquire image" {
                n139 = case shown="False" w396 {
                  tunnel: [string[] ["Cam Acq"] string[] ["Hardware reset", "Software reset", "Cam Exit", ""]] -> w400
                  frame False {
                  }
                  frame True {
                  }
                }
                n140 = for {
                  shift-right: [w406] -> w398
                  shift-left: w399 -> [w407]
                  tunnel: w400 -> [w405] mode=indexing
                  n141 = Enqueue Element(queue=w407, element=w405) -> (queue out=w406:refnum<queue>)  [unwired: 2 in, 2 out]
                }
                n142 = Select(t=TLB_MHL_States."Idle" ("Enum"), s=w396, f=TLB_MHL_States."Acquire image" ("Enum")) -> (s? t:f=w397:T6)
              }
              frame "Processing" {
              }
              frame "Shutdown" {
                # ">>State Logic >>"
                n143 = for {
                  shift-right: [w415] -> w410
                  shift-left: w411 -> [w416]
                  tunnel: string[] ["Software reset", "Hardware reset", "Motor Control", "Cam Exit", "Pre-Exit", "Exit"] -> [w414] mode=indexing
                  n144 = Enqueue Element(queue=w416, element=w414) -> (queue out=w415:refnum<queue>)  [unwired: 2 in, 2 out]
                }
              }
              frame "None" {
              }
            }
          }
        }
        "Main Loop" <- w155
      }
      n145 = while {
        tunnel: w28 -> [w652]
        tunnel: w29 -> [w651]
        tunnel: [w650] -> w35
        tunnel: [w649] -> w34
        tunnel: w33 -> [w648]
        tunnel: [w647] -> w31
        tunnel: w32 -> [w646]
        tunnel: [w645] -> w30
        i -> [w640]
        stop <- w641 stop-if-true
        # "Generate USER Event Loop"
        n146 = case shown="True" "Start Task" {
          selector: "Start Task" -> [_ w664]
          tunnel: w652 -> [w663 w668]
          tunnel: [w663 w667] -> w649
          tunnel: w648 -> [w662 w666]
          tunnel: [w662 w665] -> w647
          frame False {
          }
          frame True {
            n147 = Generate User Event(user event=w668, event data cluster=w664, error in=w666) -> (user event out=w667:refnum<user-event>, error out=w665:errorcluster)  [unwired: 1 in]
          }
        }
        n148 = case shown="False" "Stop Queue" {
          selector: "Stop Queue" -> [_ w657]
          tunnel: w651 -> [w656 w661]
          tunnel: [w656 w660] -> w650
          tunnel: w646 -> [w655 w659]
          tunnel: [w655 w658] -> w645
          tunnel: [FALSE w657] -> w641
          frame False {
          }
          frame True {
            n149 = Generate User Event(user event=w661, event data cluster=w657, error in=w659) -> (user event out=w660:refnum<user-event>, error out=w658:errorcluster)  [unwired: 1 in]
          }
        }
        n150 = call "FGV Bool.vi"("Init/Read/Write State"=States_for_Action_Engine."Write", "Input Node"=w641) -> ()  [unwired: 1 in, 2 out]
        n151 = Wait (ms)(milliseconds to wait=u32 20) -> ()  [unwired: 1 out]
        "User event loop" <- w640
      }
      n152 = while {
        i -> [w122]
        stop <- w134 stop-if-true
        w124 = 50 ("sample length")
        w139 = T20 [enum."A/AI0"] items=["Not Connected", "AudioIn/Left", "AudioIn/Right", "C/AI0", "C/AI1", "A/AI0", "A/AI1", "A/AI2", "A/AI3", "A/AI4", "A/AI5", "A/AI6", "A/AI7", "B/AI0", "B/AI1", "B/AI2", "B/AI3", "B/AI4", "B/AI5", "B/AI6", "B/AI7", "AI/AI0", "AI/AI1", "AI/AI2", "AI/AI3", "A/AI0 (DIFF)", "A/AI1 (DIFF)", "A/AI2 (DIFF)", "A/AI3 (DIFF)", "B/AI0 (DIFF)", "B/AI1 (DIFF)", "B/AI2 (DIFF)", "B/AI3 (DIFF)"] ("AI Channel")
        w140 = T20 [enum."B/AI0"] items=["Not Connected", "AudioIn/Left", "AudioIn/Right", "C/AI0", "C/AI1", "A/AI0", "A/AI1", "A/AI2", "A/AI3", "A/AI4", "A/AI5", "A/AI6", "A/AI7", "B/AI0", "B/AI1", "B/AI2", "B/AI3", "B/AI4", "B/AI5", "B/AI6", "B/AI7", "AI/AI0", "AI/AI1", "AI/AI2", "AI/AI3", "A/AI0 (DIFF)", "A/AI1 (DIFF)", "A/AI2 (DIFF)", "A/AI3 (DIFF)", "B/AI0 (DIFF)", "B/AI1 (DIFF)", "B/AI2 (DIFF)", "B/AI3 (DIFF)"] ("AI Channel")
        # "IR + Ultrasonic Sensor Loop"
        n153 = call <vilib>:"Ping.vi"("Mxp Side"=Mxp_Selection."MXP B") -> ("CM"=w128:fxp<+,64,16>)  [unwired: 8 in, 2 out]
        "Right Ultrasonic" <- w128
        "Waveform Chart 2" <- w128
        n154 = call <vilib>:"Ping.vi"("Mxp Side"=Mxp_Selection."MXP A") -> ("CM"=w129:fxp<+,64,16>)  [unwired: 8 in, 2 out]
        "Left Ultrasonic" <- w129
        "Waveform Chart" <- w129
        n155 = call <vilib>:"Sharp IR.vi"("AI Channel"=w140) -> ("Sharp IR Distance"=→"Right IR Sensor":dbl)  [unwired: 8 in, 2 out]
        n156 = call <vilib>:"Sharp IR.vi"("AI Channel"=w139) -> ("Sharp IR Distance"=→"Left IR Sensor":dbl)  [unwired: 8 in, 2 out]
        n157 = Add(x=w129, y=w128) -> (x+y=w131:fxp<+,64,17>)
        n158 = Divide(x=w131, y=fxp<+,64,17> 2.0) -> (x/y=w127:fxp<+,64,64>)
        n159 = call "FGV Bool.vi"("Init/Read/Write State"=States_for_Action_Engine."Read") -> ("Output node"=w134:bool)  [unwired: 2 in, 1 out]
        n160 = call <vilib>:"Median PtByPt.vi"("sample length"=w124, "x"=w127) -> ("median"=w126:dbl)  [unwired: 2 in, 1 out]
        n161 = call <vilib>:"Mode PtByPt.vi"("sample length"=w124, "intervals"=50, "x"=w126) -> ("mode"=→"L/R average" →"Waveform Chart 3":dbl)  [unwired: 1 in, 1 out]
        n162 = Wait Until Next ms Multiple(millisecond multiple=u32 20) -> ()  [unwired: 1 out]
        "Sensor Loop" <- w122
      }
      n163 = while {
        tunnel: w14 -> [w150]
        tunnel: w13 -> [w147]
        i -> [w141]
        stop <- w144 stop-if-true
        # "Status Loop for Action Queues"
        n164 = Get Queue Status(queue=w150, return elements? (F)=TRUE) -> (error out=w146:errorcluster, # elements in queue=→"Action Queue Items":i32, elements=→"Action Queues items":string[])  [unwired: 1 in, 5 out]
        n165 = Get Queue Status(queue=w147, return elements? (F)=TRUE) -> (# pending remove=→"State Logic Queue Items":i32, error out=w145:errorcluster)  [unwired: 1 in, 6 out]
        n166 = Merge Errors(w146, w145) -> (w144:errorcluster)
        n167 = Wait (ms)(milliseconds to wait=u32 500) -> ()  [unwired: 1 out]
        "Status loop" <- w141
      }
      n168 = while {
        tunnel: w27 -> [w613]
        tunnel: [w612] -> w26
        tunnel: w13 -> [w610]
        tunnel: [w609] -> w25
        tunnel: w19 -> [w608]
        tunnel: [w607] -> w16
        i -> [w606]
        stop <- w611 stop-if-true
        # "EVENT Handling Loop"
        n169 = event shown="[2] <Stop Queue>: User Event" {
          selector: w613 -> [_ _ _]
          dyn-events: [_ _ _] -> w612
          timeout: _ -> [_ _ _]
          tunnel: [FALSE FALSE w639] -> w611
          tunnel: w610 -> [w618 w625 w637]
          tunnel: [w617 w624 w638] -> w609
          tunnel: w608 -> [w615 w621 w635]
          tunnel: [w614 w620 w634] -> w607
          event Timeout {
            n170 = event-data() -> ()  [unwired: 1 in, 3 out]
            n171 = Enqueue Element(queue=w618, element=TLB_event_states."Idle" ("Enum"), error in (no error)=w615) -> (queue out=w617:refnum<queue>, error out=w614:errorcluster)  [unwired: 1 in, 1 out]
          }
          event User Event {
            n172 = event-data() -> ()  [unwired: 1 in, 5 out]
            n173 = case shown="\"RT Camera tracking\"" "Tasks Selector" {
              tunnel: [TLB_event_states."Idle" ("Enum") TLB_event_states."Start Task 1" ("Enum") TLB_event_states."Start Task 2" ("Enum") TLB_event_states."Start Task 3" ("Enum") TLB_event_states."Start Task 4" ("Enum") TLB_event_states."Wall follow mode" ("Enum") TLB_event_states."Camera vision" ("Enum")] -> w622
              frame Default {
              }
              frame "Task 1" {
              }
              frame "Task 2" {
              }
              frame "Task 3" {
              }
              frame "Task 4" {
              }
              frame "Wall following" {
              }
              frame "RT Camera tracking" {
              }
            }
            n174 = Enqueue Element(queue=w625, element=w622, error in (no error)=w621) -> (queue out=w624:refnum<queue>, error out=w620:errorcluster)  [unwired: 1 in, 1 out]
          }
          event User Event {
            n175 = event-data() -> ("Stop Queue"=w639:bool)  [unwired: 1 in, 4 out]
            n176 = Enqueue Element At Opposite End(queue=w637, element=TLB_event_states."Exit" ("Enum"), error in (no error)=w635) -> (queue out=w638:refnum<queue>, error out=w634:errorcluster)  [unwired: 1 in, 1 out]
          }
        }
        "Event handling loop" <- w606
      }
      n177 = while {
        i -> [w84]
        stop <- w95 stop-if-true
        (unwired) enum8{"Relay 0", "Relay 1", "Relay 2"}."Relay 0" ("Relay")
        # "Blackhawk interfacing"
        n178 = call <vilib>:"Blackhawk i2c Open.vi"("I2C Channel"=I2C_Channel."B") -> ("I2C Ref Out"=w101:T22, "error out"=w100:errorcluster)  [unwired: 2 in]
        n179 = call <vilib>:"Blackhawk DIO Read.vi"("I2C Ref In"=w101, "PIN"=u8 0, "error in (no error)"=w100) -> ("I2C Ref Out"=w93:T22, "Value Read"=→"Value Read":bool, "error out"=w94:errorcluster)  [unwired: 3 in]
        n180 = call <vilib>:"Blackhawk Relay.vi"("error in (no error)"=w94, "On/Off"="On/Off", "Relay"=enum8{"Relay 0", "Relay 1", "Relay 2"}."Relay 0", "I2C Ref In"=w93) -> ("error out"=w90:errorcluster, "I2C Ref Out"=w86:T22)  [unwired: 6 in]
        n181 = call <vilib>:"Blackhawk Servo.vi"("error in (no error)"=w90, "Servo Select"=enum16{"Servo 5", "Servo 6"}."Servo 5", "Servo Angle"="Servo Angle", "I2C Ref In"=w86) -> ("error out"=→"Blackhawk error":errorcluster)  [unwired: 6 in, 1 out]
        n182 = call "FGV Bool.vi"("Init/Read/Write State"=States_for_Action_Engine."Read") -> ("Output node"=w95:bool)  [unwired: 2 in, 1 out]
        n183 = Wait (ms)(milliseconds to wait=u32 20) -> ()  [unwired: 1 out]
        "Blackhawk loop" <- w84
      }
      n184 = while {
        tunnel: [w114] -> w7
        tunnel: [w111] -> w6
        tunnel: [w110] -> w4
        tunnel: [w109] -> w5
        tunnel: [w108] -> w3
        i -> [w102]
        stop <- w116 stop-if-true
        # "NavX Loop"
        n185 = call <vilib>:"NavX Open.vi"("I2C Channel"=I2C_Channel."A") -> ("NavX Info"=w103:T8)  [unwired: 9 in, 1 out]
        n186 = case shown="True" "NavX Zero Yaw" {
          tunnel: w103 -> [w118 w120]
          tunnel: [w118 w119] -> w108
          frame False {
          }
          frame True {
            n187 = call <vilib>:"Zero Yaw.vi"("NavX Info In"=w120) -> ("NavX Info Out"=w119:T8)  [unwired: 10 in]
          }
        }
        n188 = call <vilib>:"YRPHfH.vi"("NavX Info In"=w103) -> ("YRPHfH"=w106:T11, "NavX Info Out"=w110:T8)  [unwired: 3 in]
        "YRPHfH" <- w106
        n189 = call <vilib>:"Raw Values.vi"("NavX Info In"=w103) -> ("NavX Info Out"=w114:T8)  [unwired: 8 in, 1 out]
        "NavX Info Out" <- w114
        n190 = call <vilib>:"LinearAcceleration.vi"("NavX Info In"=w103) -> ("LinearAcceleration"=→"LinearAcceleration":T9, "NavX Info Out"=w111:T8)  [unwired: 9 in]
        n191 = call <vilib>:"Displacement.vi"("NavX Info In"=w103) -> ("Displacement"=→"Displacement":T10, "NavX Info Out"=w109:T8)  [unwired: 9 in]
        n192 = Unbundle By Name(w106) -> ("Yaw"=→"Yaw":dbl)
        n193 = call "FGV Bool.vi"("Init/Read/Write State"=States_for_Action_Engine."Read") -> ("Output node"=w116:bool)  [unwired: 2 in, 1 out]
        n194 = Wait Until Next ms Multiple(millisecond multiple=u32 10) -> ()  [unwired: 1 out]
        "NavX Loop" <- w102
      }
      n195 = disable-structure shown="Disabled" {
        frame Disabled {
          n196 = call <vilib>:"IMAQdx Open Camera.vi"("Session In"=T16 "cam1") -> ("error out"=w51:errorcluster, "Session Out"=w53:T16)  [unwired: 9 in]
          n197 = call "IMAQ Create"("Image Name"="image") -> ("New Image"=w66:T4, "error out"=w65:errorcluster)  [unwired: 4 in]
          n198 = call <vilib>:"IMAQdx Configure Acquisition.vi"("error in"=w51, "Number of Buffers"=u32 1, "Continuous?"=IMAQdx_Acquisition_Mode."Continuous", "Session In"=w53) -> ("error out"=w50:errorcluster, "Session Out"=w52:T16)  [unwired: 6 in]
          n199 = call <vilib>:"IMAQdx Start Acquisition.vi"("error in"=w50, "Session In"=w52) -> ("error out"=w60:errorcluster, "Session Out"=w61:T16)  [unwired: 8 in]
          n200 = while {
            tunnel: w66 -> [w75]
            tunnel: w65 -> [w79]
            tunnel: [w75] -> w64
            tunnel: [w78] -> w63
            tunnel: [w78] -> w55
            tunnel: w61 -> [w77]
            tunnel: w60 -> [w76]
            tunnel: [w73] -> w54
            stop <- w81 stop-if-true
            # "Webcam loop"
            n201 = call <vilib>:"IMAQdx Get Image2.vi"("Buffer Number Mode (Next)"=IMAQdx_Buffer_Number_Mode."Next", "error in"=w76, "Image In"=w75, "Session In"=w77) -> ("error out"=w70:errorcluster, "Image Out"=w71:T4, "Session Out"=w73:T16)  [unwired: 4 in, 1 out]
            n202 = Wait (ms)(milliseconds to wait=u32 500) -> ()  [unwired: 1 out]
            n203 = call "All object detection ver2.vi"("error in"=w70, "Image In"=w71) -> ("error out"=w72:errorcluster, "Image Out"=w68:T4)
            n204 = case shown="True" w69 {
              tunnel: [_ w83] -> _
              tunnel: w68 -> [_ w83]
              frame False {
              }
              frame True {
              }
            }
            n205 = Merge Errors(w72, w79) -> (w78:errorcluster)
            n206 = call "FGV Bool.vi"("Init/Read/Write State"=States_for_Action_Engine."Read") -> ("Output node"=w81:bool)  [unwired: 2 in, 1 out]
          }
          n207 = call "Imaq Dispose"("All Images? (No)"=TRUE, "Image"=w64, "error in (no error)"=w63) -> ()  [unwired: 3 in, 1 out]
          n208 = call <vilib>:"IMAQdx Stop Acquisition.vi"("error in"=w55, "Session In"=w54) -> ("error out"=w58:errorcluster, "Session Out"=w59:T16)  [unwired: 8 in]
          n209 = call <vilib>:"IMAQdx Unconfigure Acquisition.vi"("error in"=w58, "Session In"=w59) -> ("error out"=w56:errorcluster, "Session Out"=w57:T16)  [unwired: 8 in]
          n210 = call <vilib>:"IMAQdx Close Camera.vi"("error in"=w56, "Session In"=w57) -> ()  [unwired: 9 in, 1 out]
        }
        frame Enabled {
        }
      }
      n211 = while {
        stop <- w39 stop-if-true
        n212 = Wait Until Next ms Multiple(millisecond multiple=u32 5) -> ()  [unwired: 1 out]
        n213 = call "New motor Control integrated.vi"("wTargetSpeed"="wTargetSpeed", "yTargetSpeed"="yTargetSpeed", "xTargetSpeed"="xTargetSpeed", "Reset Encoders"="Reset Encoders") -> ("Speed"=→"Speed":T1, "Distance"=→"Distance":T2)
        n214 = call "FGV Bool.vi"("Init/Read/Write State"=States_for_Action_Engine."Read") -> ("Output node"=w39:bool)  [unwired: 2 in, 1 out]
      }
      n215 = call <vilib>:"NavX Close.vi"("NavX Info In"=w3) -> ()  [unwired: 10 in, 1 out]
      n216 = call <vilib>:"NavX Close.vi"("NavX Info In"=w7) -> ()  [unwired: 10 in, 1 out]
      n217 = call <vilib>:"NavX Close.vi"("NavX Info In"=w6) -> ()  [unwired: 10 in, 1 out]
      n218 = call <vilib>:"NavX Close.vi"("NavX Info In"=w5) -> ()  [unwired: 10 in, 1 out]
      n219 = call <vilib>:"NavX Close.vi"("NavX Info In"=w4) -> ()  [unwired: 10 in, 1 out]
      n220 = Merge Errors "Merge Errors"(w31, w30) -> (w10:errorcluster)
      n221 = Merge Errors(w16, w10) -> (w12:errorcluster)
      n222 = Destroy User Event(user event=w34, error in=w12) -> ()  [unwired: 1 out]
      n223 = Destroy User Event(user event=w35, error in=w12) -> ()  [unwired: 1 out]
      n224 = Unregister For Events(event registration refnum=w26, error in=w12) -> ()  [unwired: 1 out]
      n225 = Release Queue(queue=w25, error in (no error)=w12) -> ()  [unwired: 1 in, 3 out]
      n226 = Release Queue(queue=w11, error in (no error)=w12) -> ()  [unwired: 1 in, 3 out]
    }
    frame #2 {
    }
  }
